vi "Add Node.vi"(8 "error in (no error)":errorcluster, 10 "Node to Add":refnum<class "INode.lvclass">, 11 "node in":refnum<class "node.lvclass">) -> (0 "error out":errorcluster, 3 "node out":refnum<class "node.lvclass">)   [LabVIEW 2021, in "d7.lvlib" / "node.lvclass"]
uses:
  node.lvclass
  INode/INode.lvclass
  node.lvclass/node.ctl
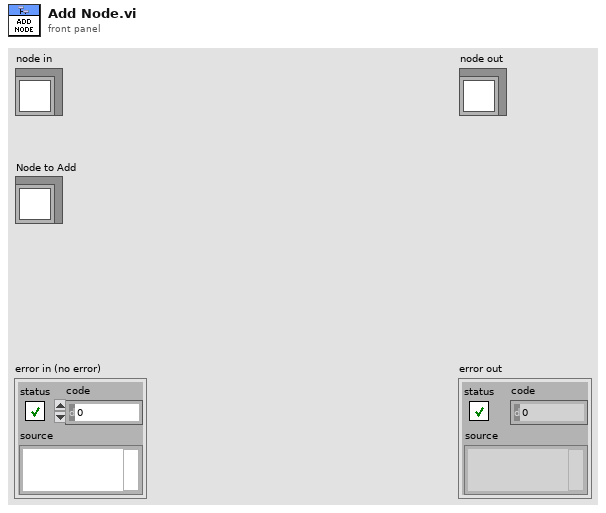
[diagram p1: front panel]
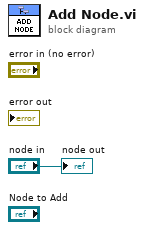
[diagram p0: block diagram]
diagram:
  "node out" <- "node in"
